vi "toVariant.vi"(2 "data type":T1, 3 "value":u8[](array[numeric]), 4 "dim. y":i32, 5 "dim. x":i32) -> (0 "Setpoint":variant, 1 "Value":variant)   [LabVIEW 2014, in "tango.lvlib"]
uses:
  tango.lvlib
  toStateScalar.vi
  toStateSpectrum.vi
  toStateImage.vi
  toStringScalar.vi
  toStringSpectrum.vi
  toStringImage.vi
  toBooleanScalar.vi
  toBooleanSpectrum.vi
  toBooleanImage.vi
  toUCharScalar.vi
  toUCharSpectrum.vi
  toUCharImage.vi
  toShortScalar.vi
  toShortSpectrum.vi
  toShortImage.vi
  toUShortScalar.vi
  toUShortSpectrum.vi
  toUShortImage.vi
  toLongScalar.vi
  toLongSpectrum.vi
  toLongImage.vi
  toULongScalar.vi
  toULongSpectrum.vi
  toULongImage.vi
  toLong64Scalar.vi
  toLong64Spectrum.vi
  toLong64mage.vi
  toULong64Scalar.vi
  toULong64Spectrum.vi
  toULong64Image.vi
  toFloatScalar.vi
  toFloatSpectrum.vi
  toFloatImage.vi
  toDoubleScalar.vi
  toDoubleSpectrum.vi
  toDoubleImage.vi
  Common VIs/Typedefs/_AttributeDataType_t.ctl
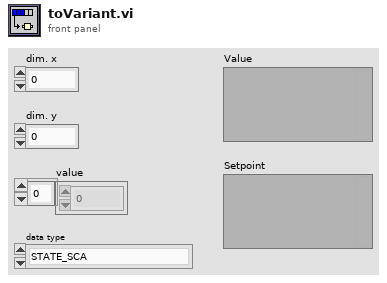
[diagram p1: front panel]
types:
  T1 = typedef "tango.lvlib/_AttributeDataType_t.ctl" = enum16{"STATE_SCA", "STATE_SPE", "STATE_IMG", "STRING_SCA", "STRING_SPE", "STRING_IMG", "BOOL_SCA", "BOOL_SPE", "BOOL_IMG", "UCHAR_SCA", "UCHAR_SPE", "UCHAR_IMG", "SHORT_SCA", "SHORT_SPE", "SHORT_IMG", "USHORT_SCA", "USHORT_SPE", "USHORT_IMG", "LONG_SCA", "LONG_SPE", "LONG_IMG", "ULONG_SCA", "ULONG_SPE", "ULONG_IMG", "LONG64_SCA", "LONG64_SPE", "LONG64_IMG", "ULONG64_SCA", "ULONG64_SPE", "ULONG64_IMG", "FLOAT_SCA", "FLOAT_SPE", "FLOAT_IMG", "DOUBLE_SCA", "DOUBLE_SPE", "DOUBLE_IMG", "ENUM_SCA", "UNKNOWN_DATA_TYPE"}
  T2 = typedef "tango.lvlib/_TangoState_t.ctl" = enum32{"ON", "OFF", "CLOSE", "OPEN", "INSERT", "EXTRACT", "MOVING", "STANDBY", "FAULT", "INIT", "RUNNING", "ALARM", "DISABLE", "UNKNOWN"}
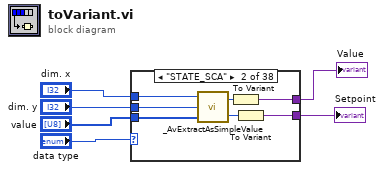
[diagram p0: block diagram]
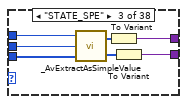
[diagram p3: hidden frame]
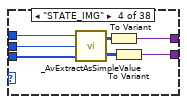
[diagram p4: hidden frame]
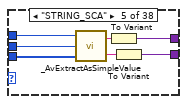
[diagram p5: hidden frame]
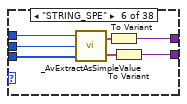
[diagram p6: hidden frame]
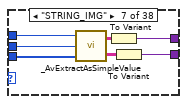
[diagram p7: hidden frame]
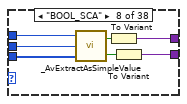
[diagram p8: hidden frame]
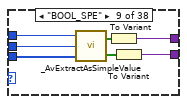
[diagram p9: hidden frame]
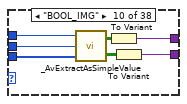
[diagram p10: hidden frame]
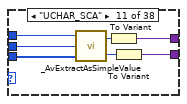
[diagram p11: hidden frame]
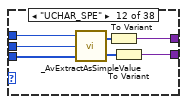
[diagram p12: hidden frame]
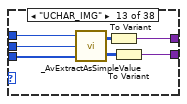
[diagram p13: hidden frame]
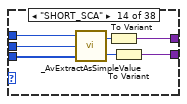
[diagram p14: hidden frame]
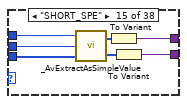
[diagram p15: hidden frame]
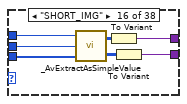
[diagram p16: hidden frame]
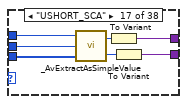
[diagram p17: hidden frame]
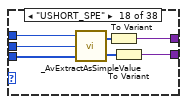
[diagram p18: hidden frame]
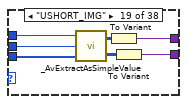
[diagram p19: hidden frame]
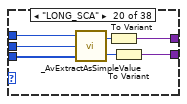
[diagram p20: hidden frame]
diagram:
  n1 = case shown="\"STATE_SCA\"" "data type" {
    tunnel: "value" -> [_ w13 w20 w27 w34 w41 w48 w55 w62 w69 w76 w83 w90 w97 w104 w111 w118 w125 w132 w139 w146 w153 w160 w167 w174 w181 w188 w195 w202 w209 w216 w223 w230 w237 w244 w251 w258 _]
    tunnel: "dim. y" -> [_ w12 w19 w26 w33 w40 w47 w54 w61 w68 w75 w82 w89 w96 w103 w110 w117 w124 w131 w138 w145 w152 w159 w166 w173 w180 w187 w194 w201 w208 w215 w222 w229 w236 w243 w250 w257 _]
    tunnel: "dim. x" -> [_ w11 w18 w25 w32 w39 w46 w53 w60 w67 w74 w81 w88 w95 w102 w109 w116 w123 w130 w137 w144 w151 w158 w165 w172 w179 w186 w193 w200 w207 w214 w221 w228 w235 w242 w249 w256 _]
    tunnel: [_ w8 w15 w22 w29 w36 w43 w50 w57 w64 w71 w78 w85 w92 w99 w106 w113 w120 w127 w134 w141 w148 w155 w162 w169 w176 w183 w190 w197 w204 w211 w218 w225 w232 w239 w246 w253 _] -> w4
    tunnel: [_ w7 w14 w21 w28 w35 w42 w49 w56 w63 w70 w77 w84 w91 w98 w105 w112 w119 w126 w133 w140 w147 w154 w161 w168 w175 w182 w189 w196 w203 w210 w217 w224 w231 w238 w245 w252 _] -> w5
    frame "UNKNOWN_DATA_TYPE", Default {
    }
    frame "STATE_SCA" {
      n2 = call-poly "_AvExtractAsSimpleValue.vi"("value_in"=w13, "dim_y"=w12, "dim_x"=w11) -> ("setpoint"=w9:T2, "value_out"=w10:T2)
      n3 = To Variant(anything=w10) -> (Variant=w8:variant)
      n4 = To Variant(anything=w9) -> (Variant=w7:variant)
    }
    frame "STATE_SPE" {
      n5 = call-poly "_AvExtractAsSimpleValue.vi"("value_in"=w20, "dim_y"=w19, "dim_x"=w18) -> ("setpoint"=w16:T2[], "value_out"=w17:T2[])
      n6 = To Variant(anything=w17) -> (Variant=w15:variant)
      n7 = To Variant(anything=w16) -> (Variant=w14:variant)
    }
    frame "STATE_IMG" {
      n8 = call-poly "_AvExtractAsSimpleValue.vi"("value_in"=w27, "dim_y"=w26, "dim_x"=w25) -> ("setpoint"=w23:T2[][], "value_out"=w24:T2[][])
      n9 = To Variant(anything=w24) -> (Variant=w22:variant)
      n10 = To Variant(anything=w23) -> (Variant=w21:variant)
    }
    frame "STRING_SCA" {
      n11 = call-poly "_AvExtractAsSimpleValue.vi"("value_in"=w34, "dim_y"=w33, "dim_x"=w32) -> ("setpoint"=w30:string, "value_out"=w31:string)
      n12 = To Variant(anything=w31) -> (Variant=w29:variant)
      n13 = To Variant(anything=w30) -> (Variant=w28:variant)
    }
    frame "STRING_SPE" {
      n14 = call-poly "_AvExtractAsSimpleValue.vi"("value_in"=w41, "dim_y"=w40, "dim_x"=w39) -> ("setpoint"=w37:string[], "value_out"=w38:string[])
      n15 = To Variant(anything=w38) -> (Variant=w36:variant)
      n16 = To Variant(anything=w37) -> (Variant=w35:variant)
    }
    frame "STRING_IMG" {
      n17 = call-poly "_AvExtractAsSimpleValue.vi"("value_in"=w48, "dim_y"=w47, "dim_x"=w46) -> ("setpoint"=w44:string[][], "value_out"=w45:string[][])
      n18 = To Variant(anything=w45) -> (Variant=w43:variant)
      n19 = To Variant(anything=w44) -> (Variant=w42:variant)
    }
    frame "BOOL_SCA" {
      n20 = call-poly "_AvExtractAsSimpleValue.vi"("value_in"=w55, "dim_y"=w54, "dim_x"=w53) -> ("setpoint"=w51:bool, "value_out"=w52:bool)
      n21 = To Variant(anything=w52) -> (Variant=w50:variant)
      n22 = To Variant(anything=w51) -> (Variant=w49:variant)
    }
    frame "BOOL_SPE" {
      n23 = call-poly "_AvExtractAsSimpleValue.vi"("value_in"=w62, "dim_y"=w61, "dim_x"=w60) -> ("setpoint"=w58:bool[], "value_out"=w59:bool[])
      n24 = To Variant(anything=w59) -> (Variant=w57:variant)
      n25 = To Variant(anything=w58) -> (Variant=w56:variant)
    }
    frame "BOOL_IMG" {
      n26 = call-poly "_AvExtractAsSimpleValue.vi"("value_in"=w69, "dim_y"=w68, "dim_x"=w67) -> ("setpoint"=w65:bool[][], "value_out"=w66:bool[][])
      n27 = To Variant(anything=w66) -> (Variant=w64:variant)
      n28 = To Variant(anything=w65) -> (Variant=w63:variant)
    }
    frame "UCHAR_SCA" {
      n29 = call-poly "_AvExtractAsSimpleValue.vi"("value_in"=w76, "dim_y"=w75, "dim_x"=w74) -> ("setpoint"=w72:u8, "value_out"=w73:u8)
      n30 = To Variant(anything=w73) -> (Variant=w71:variant)
      n31 = To Variant(anything=w72) -> (Variant=w70:variant)
    }
    frame "UCHAR_SPE" {
      n32 = call-poly "_AvExtractAsSimpleValue.vi"("value_in"=w83, "dim_y"=w82, "dim_x"=w81) -> ("setpoint"=w79:u8[], "value_out"=w80:u8[])
      n33 = To Variant(anything=w80) -> (Variant=w78:variant)
      n34 = To Variant(anything=w79) -> (Variant=w77:variant)
    }
    frame "UCHAR_IMG" {
      n35 = call-poly "_AvExtractAsSimpleValue.vi"("value_in"=w90, "dim_y"=w89, "dim_x"=w88) -> ("setpoint"=w86:u8[][], "value_out"=w87:u8[][])
      n36 = To Variant(anything=w87) -> (Variant=w85:variant)
      n37 = To Variant(anything=w86) -> (Variant=w84:variant)
    }
    frame "SHORT_SCA" {
      n38 = call-poly "_AvExtractAsSimpleValue.vi"("value_in"=w97, "dim_y"=w96, "dim_x"=w95) -> ("setpoint"=w93:i16, "value_out"=w94:i16)
      n39 = To Variant(anything=w94) -> (Variant=w92:variant)
      n40 = To Variant(anything=w93) -> (Variant=w91:variant)
    }
    frame "SHORT_SPE" {
      n41 = call-poly "_AvExtractAsSimpleValue.vi"("value_in"=w104, "dim_y"=w103, "dim_x"=w102) -> ("setpoint"=w100:i16[], "value_out"=w101:i16[])
      n42 = To Variant(anything=w101) -> (Variant=w99:variant)
      n43 = To Variant(anything=w100) -> (Variant=w98:variant)
    }
    frame "SHORT_IMG" {
      n44 = call-poly "_AvExtractAsSimpleValue.vi"("value_in"=w111, "dim_y"=w110, "dim_x"=w109) -> ("setpoint"=w107:i16[][], "value_out"=w108:i16[][])
      n45 = To Variant(anything=w108) -> (Variant=w106:variant)
      n46 = To Variant(anything=w107) -> (Variant=w105:variant)
    }
    frame "USHORT_SCA" {
      n47 = call-poly "_AvExtractAsSimpleValue.vi"("value_in"=w118, "dim_y"=w117, "dim_x"=w116) -> ("setpoint"=w114:u16, "value_out"=w115:u16)
      n48 = To Variant(anything=w115) -> (Variant=w113:variant)
      n49 = To Variant(anything=w114) -> (Variant=w112:variant)
    }
    frame "USHORT_SPE" {
      n50 = call-poly "_AvExtractAsSimpleValue.vi"("value_in"=w125, "dim_y"=w124, "dim_x"=w123) -> ("setpoint"=w121:u16[], "value_out"=w122:u16[])
      n51 = To Variant(anything=w122) -> (Variant=w120:variant)
      n52 = To Variant(anything=w121) -> (Variant=w119:variant)
    }
    frame "USHORT_IMG" {
      n53 = call-poly "_AvExtractAsSimpleValue.vi"("value_in"=w132, "dim_y"=w131, "dim_x"=w130) -> ("setpoint"=w128:u16[][], "value_out"=w129:u16[][])
      n54 = To Variant(anything=w129) -> (Variant=w127:variant)
      n55 = To Variant(anything=w128) -> (Variant=w126:variant)
    }
    frame "LONG_SCA" {
      n56 = call-poly "_AvExtractAsSimpleValue.vi"("value_in"=w139, "dim_y"=w138, "dim_x"=w137) -> ("setpoint"=w135:i32, "value_out"=w136:i32)
      n57 = To Variant(anything=w136) -> (Variant=w134:variant)
      n58 = To Variant(anything=w135) -> (Variant=w133:variant)
    }
    frame "LONG_SPE" {
      n59 = call-poly "_AvExtractAsSimpleValue.vi"("value_in"=w146, "dim_y"=w145, "dim_x"=w144) -> ("setpoint"=w142:i32[], "value_out"=w143:i32[])
      n60 = To Variant(anything=w143) -> (Variant=w141:variant)
      n61 = To Variant(anything=w142) -> (Variant=w140:variant)
    }
    frame "LONG_IMG" {
      n62 = call-poly "_AvExtractAsSimpleValue.vi"("value_in"=w153, "dim_y"=w152, "dim_x"=w151) -> ("setpoint"=w149:i32[][], "value_out"=w150:i32[][])
      n63 = To Variant(anything=w150) -> (Variant=w148:variant)
      n64 = To Variant(anything=w149) -> (Variant=w147:variant)
    }
    frame "ULONG_SCA" {
      n65 = call-poly "_AvExtractAsSimpleValue.vi"("value_in"=w160, "dim_y"=w159, "dim_x"=w158) -> ("setpoint"=w156:u32, "value_out"=w157:u32)
      n66 = To Variant(anything=w157) -> (Variant=w155:variant)
      n67 = To Variant(anything=w156) -> (Variant=w154:variant)
    }
    frame "ULONG_SPE" {
      n68 = call-poly "_AvExtractAsSimpleValue.vi"("value_in"=w167, "dim_y"=w166, "dim_x"=w165) -> ("setpoint"=w163:u32[], "value_out"=w164:u32[])
      n69 = To Variant(anything=w164) -> (Variant=w162:variant)
      n70 = To Variant(anything=w163) -> (Variant=w161:variant)
    }
    frame "ULONG_IMG" {
      n71 = call-poly "_AvExtractAsSimpleValue.vi"("value_in"=w174, "dim_y"=w173, "dim_x"=w172) -> ("setpoint"=w170:u32[][], "value_out"=w171:u32[][])
      n72 = To Variant(anything=w171) -> (Variant=w169:variant)
      n73 = To Variant(anything=w170) -> (Variant=w168:variant)
    }
    frame "LONG64_SCA" {
      n74 = call-poly "_AvExtractAsSimpleValue.vi"("value_in"=w181, "dim_y"=w180, "dim_x"=w179) -> ("setpoint"=w177:i64, "value"=w178:i64)
      n75 = To Variant(anything=w178) -> (Variant=w176:variant)
      n76 = To Variant(anything=w177) -> (Variant=w175:variant)
    }
    frame "LONG64_SPE" {
      n77 = call-poly "_AvExtractAsSimpleValue.vi"("value_in"=w188, "dim_y"=w187, "dim_x"=w186) -> ("setpoint"=w184:i64[], "value"=w185:i64[])
      n78 = To Variant(anything=w185) -> (Variant=w183:variant)
      n79 = To Variant(anything=w184) -> (Variant=w182:variant)
    }
    frame "LONG64_IMG" {
      n80 = call-poly "_AvExtractAsSimpleValue.vi"("value_in"=w195, "dim_y"=w194, "dim_x"=w193) -> ("setpoint"=w191:i64[][], "value"=w192:i64[][])
      n81 = To Variant(anything=w192) -> (Variant=w190:variant)
      n82 = To Variant(anything=w191) -> (Variant=w189:variant)
    }
    frame "ULONG64_SCA" {
      n83 = call-poly "_AvExtractAsSimpleValue.vi"("value_in"=w202, "dim_y"=w201, "dim_x"=w200) -> ("setpoint"=w198:u64, "value"=w199:u64)
      n84 = To Variant(anything=w199) -> (Variant=w197:variant)
      n85 = To Variant(anything=w198) -> (Variant=w196:variant)
    }
    frame "ULONG64_SPE" {
      n86 = call-poly "_AvExtractAsSimpleValue.vi"("value_in"=w209, "dim_y"=w208, "dim_x"=w207) -> ("setpoint"=w205:u64[], "value"=w206:u64[])
      n87 = To Variant(anything=w206) -> (Variant=w204:variant)
      n88 = To Variant(anything=w205) -> (Variant=w203:variant)
    }
    frame "ULONG64_IMG" {
      n89 = call-poly "_AvExtractAsSimpleValue.vi"("value_in"=w216, "dim_y"=w215, "dim_x"=w214) -> ("setpoint"=w212:u64[][], "value"=w213:u64[][])
      n90 = To Variant(anything=w213) -> (Variant=w211:variant)
      n91 = To Variant(anything=w212) -> (Variant=w210:variant)
    }
    frame "FLOAT_SCA" {
      n92 = call-poly "_AvExtractAsSimpleValue.vi"("value_in"=w223, "dim_y"=w222, "dim_x"=w221) -> ("setpoint"=w219:sgl, "value_out"=w220:sgl)
      n93 = To Variant(anything=w220) -> (Variant=w218:variant)
      n94 = To Variant(anything=w219) -> (Variant=w217:variant)
    }
    frame "FLOAT_SPE" {
      n95 = call-poly "_AvExtractAsSimpleValue.vi"("value_in"=w230, "dim_y"=w229, "dim_x"=w228) -> ("setpoint"=w226:sgl[], "value_out"=w227:sgl[])
      n96 = To Variant(anything=w227) -> (Variant=w225:variant)
      n97 = To Variant(anything=w226) -> (Variant=w224:variant)
    }
    frame "FLOAT_IMG" {
      n98 = call-poly "_AvExtractAsSimpleValue.vi"("value_in"=w237, "dim_y"=w236, "dim_x"=w235) -> ("setpoint"=w233:sgl[][], "value_out"=w234:sgl[][])
      n99 = To Variant(anything=w234) -> (Variant=w232:variant)
      n100 = To Variant(anything=w233) -> (Variant=w231:variant)
    }
    frame "DOUBLE_SCA" {
      n101 = call-poly "_AvExtractAsSimpleValue.vi"("value_in"=w244, "dim_y"=w243, "dim_x"=w242) -> ("setpoint"=w240:dbl, "value_out"=w241:dbl)
      n102 = To Variant(anything=w241) -> (Variant=w239:variant)
      n103 = To Variant(anything=w240) -> (Variant=w238:variant)
    }
    frame "DOUBLE_SPE" {
      n104 = call-poly "_AvExtractAsSimpleValue.vi"("value_in"=w251, "dim_y"=w250, "dim_x"=w249) -> ("setpoint"=w247:dbl[], "value_out"=w248:dbl[])
      n105 = To Variant(anything=w248) -> (Variant=w246:variant)
      n106 = To Variant(anything=w247) -> (Variant=w245:variant)
    }
    frame "DOUBLE_IMG" {
      n107 = call-poly "_AvExtractAsSimpleValue.vi"("value_in"=w258, "dim_y"=w257, "dim_x"=w256) -> ("setpoint"=w254:dbl[][], "value_out"=w255:dbl[][])
      n108 = To Variant(anything=w255) -> (Variant=w253:variant)
      n109 = To Variant(anything=w254) -> (Variant=w252:variant)
    }
    frame "ENUM_SCA" {
      # "?"
    }
  }
  "Setpoint" <- w5
  "Value" <- w4
